vi "Get_Values.vi"(0 "reference in":refnum<class "AO.lvclass">) -> ()   [LabVIEW 2019, in "AO.lvclass"]
uses:
  AO.lvclass
  AO.lvclass/AO.ctl
panel:
  out "Value":dbl
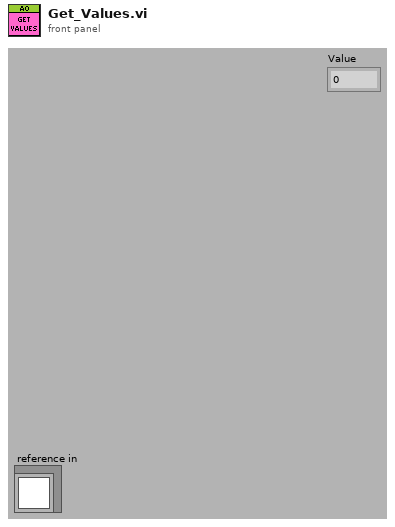
[diagram p1: front panel]
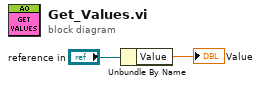
[diagram p0: block diagram]
diagram:
  n1 = Unbundle By Name("reference in") -> ("Value"=→"Value":dbl)
